vi "systemsResponseStatus.vi"   [LabVIEW 2021]
types:
  T1 = cluster{"Valve compensator HT":bool, "Valve compensator LT ":bool, "Temperature module HT":bool, "Temperature module LT":bool, "Pressure module":bool, "Power module":bool}
  T2 = cluster{"ValvePos1":sgl, "ValvePos2":sgl, "PressureArray":sgl[], "TempArray2":sgl[], "TempArray1":sgl[], "Valve 1 Time Stamp":timestamp, "Temp 2 Array Time Stamp":timestamp[], "Temp 1 Array Time Stamp":timestamp[], "Valve 2 Time Stamp":timestamp, "Press Array Time Stamp":timestamp[]}
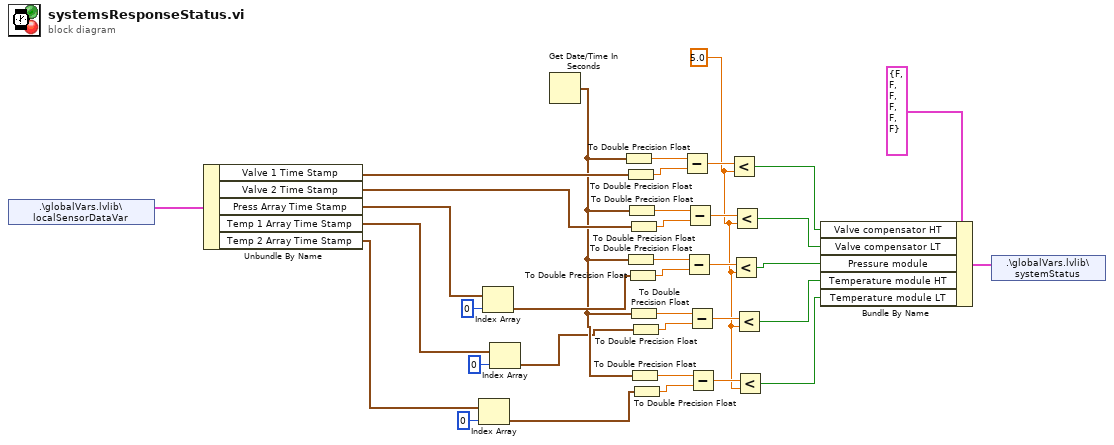
[diagram p0: block diagram]
diagram:
  w11 = 5.0
  n1 = shared-variable ".\\globalVars.lvlib\\localSensorDataVar"() -> (w36:T2)  [unwired: 1 in, 1 out]
  n2 = Unbundle By Name(w36) -> ("Valve 1 Time Stamp"=w28:timestamp, "Valve 2 Time Stamp"=w13:timestamp, "Press Array Time Stamp"=w33:timestamp[], "Temp 1 Array Time Stamp"=w35:timestamp[], "Temp 2 Array Time Stamp"=w34:timestamp[])
  n3 = Index Array(array=w34, index=0) -> (element=w12:timestamp)
  n4 = Index Array(array=w33, index=0) -> (element=w3:timestamp)
  n5 = Index Array(array=w35, index=0) -> (element=w1:timestamp)
  n6 = Get Date/Time In Seconds() -> (seconds since 1Jan1904=w2:timestamp)
  n7 = To Double Precision Float(number=w2) -> (double precision float=w29:dbl)
  n8 = To Double Precision Float(number=w28) -> (double precision float=w27:dbl)
  n9 = To Double Precision Float(number=w2) -> (double precision float=w20:dbl)
  n10 = To Double Precision Float(number=w2) -> (double precision float=w25:dbl)
  n11 = To Double Precision Float(number=w3) -> (double precision float=w21:dbl)
  n12 = To Double Precision Float(number=w13) -> (double precision float=w24:dbl)
  n13 = To Double Precision Float(number=w2) -> (double precision float=w19:dbl)
  n14 = To Double Precision Float(number=w2) -> (double precision float=w14:dbl)
  n15 = To Double Precision Float(number=w1) -> (double precision float=w18:dbl)
  n16 = To Double Precision Float(number=w12) -> (double precision float=w15:dbl)
  n17 = Subtract(x=w29, y=w27) -> (x-y=w26:dbl)
  n18 = Subtract(x=w20, y=w21) -> (x-y=w22:dbl)
  n19 = Subtract(x=w25, y=w24) -> (x-y=w23:dbl)
  n20 = Subtract(x=w19, y=w18) -> (x-y=w17:dbl)
  n21 = Subtract(x=w14, y=w15) -> (x-y=w16:dbl)
  n22 = Less?(x=w26, y=w11) -> (x < y?=w8:bool)
  n23 = Less?(x=w22, y=w11) -> (x < y?=w6:bool)
  n24 = Less?(x=w23, y=w11) -> (x < y?=w7:bool)
  n25 = Less?(x=w17, y=w11) -> (x < y?=w5:bool)
  n26 = Less?(x=w16, y=w11) -> (x < y?=w4:bool)
  n27 = Bundle By Name(cluster=T1 {"Valve compensator HT"=FALSE, "Valve compensator LT "=FALSE, "Temperature module HT"=FALSE, "Temperature module LT"=FALSE, "Pressure module"=FALSE, "Power module"=FALSE} ("systemStatus"), "Valve compensator HT"=w8, "Valve compensator LT"=w7, "Pressure module"=w6, "Temperature module HT"=w5, "Temperature module LT"=w4) -> (w9:T1)
  n28 = shared-variable ".\\globalVars.lvlib\\systemStatus"(w9) -> ()  [unwired: 1 in, 1 out]
